vi "Connect.vi"(8 "error in (no error)":errorcluster, 10 "Addon Name":string, 11 "Address":string) -> (0 "error out":errorcluster, 3 "Ref":T1)   [LabVIEW 2019, in "Diagnostics Host Automation API.lvlib"]
uses:
  Diagnostics Host Automation API.lvlib
  Addon/Addon Shared/Types/HostAutomation.Ref.ctl
  <vilib>/NI/STM/TCP/TCP Connection Info.ctl
  <vilib>/NI/STM/SubVIs/MetaDataElement.ctl
  Addon/Addon Shared/Types/DTC.Codes.ctl
  <vilib>/NI/STM/TCP/Write Meta Data (TCP Ref).vi
  <vilib>/NI/STM/TCP/Write Meta Data (TCP Clst).vi
  <vilib>/NI/STM/NI STM.lvlib
  Addon/Addon Shared/Diagnostics Addon Shared.lvlib
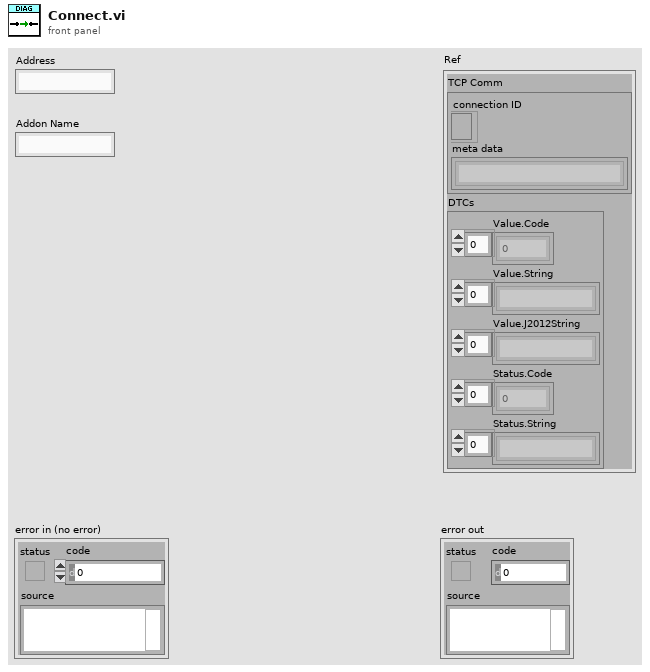
[diagram p1: front panel]
types:
  T1 = typedef "Diagnostics Addon Shared.lvlib/HostAutomation.Ref.ctl" = cluster{"TCP Comm":T2, "DTCs":T4}
  T2 = typedef "NI STM.lvlib/TCP Connection Info.ctl" = cluster{"connection ID":refnum<k5>, "meta data":T3[]}
  T3 = typedef "NI STM.lvlib/MetaDataElement.ctl" = string
  T4 = typedef "Diagnostics Addon Shared.lvlib/DTC.Codes.ctl" = cluster{"Value.Code":dbl[], "Value.String":string[], "Value.J2012String":string[], "Status.Code":dbl[], "Status.String":string[]}
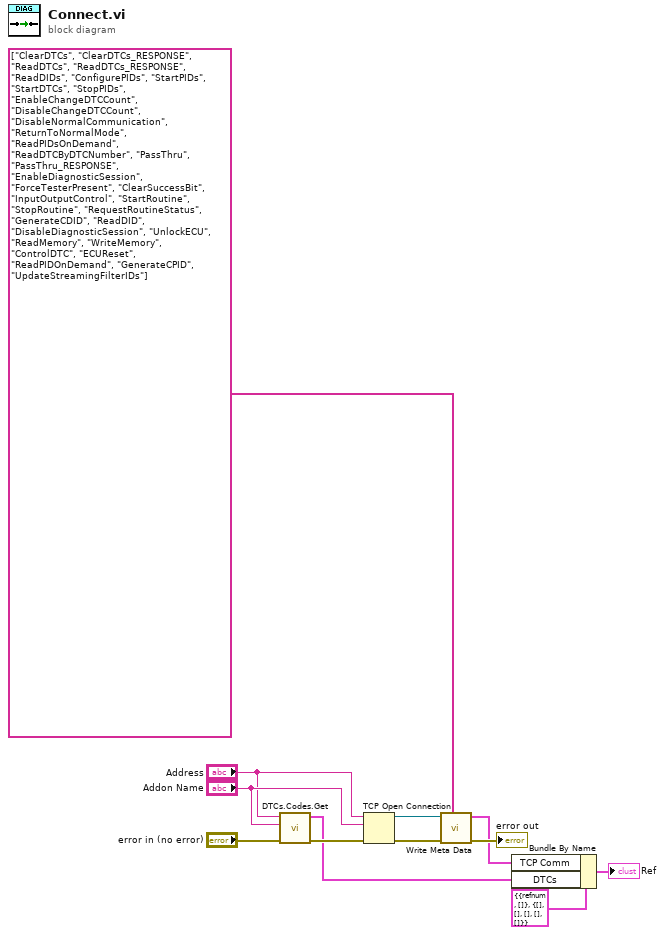
[diagram p0: block diagram]
diagram:
  n1 = call "DTCs.Codes.Get.vi"("error in (no error)"="error in (no error)", "Addon Name"="Addon Name", "Address"="Address") -> ("error out"=w6:errorcluster, "Codes"=w2:T4)  [unwired: 7 in]
  n2 = TCP Open Connection(address="Address", remote port or service name="Addon Name", error in (no error)=w6) -> (connection ID=w11:refnum<k5>, error out=w12:errorcluster)  [unwired: 2 in]
  n3 = call-poly <vilib>:"Write Meta Data.vi"("meta data"=string[] ["ClearDTCs", "ClearDTCs_RESPONSE", "ReadDTCs", "ReadDTCs_RESPONSE", "ReadDIDs", "ConfigurePIDs", "StartPIDs", "StartDTCs", "StopPIDs", "EnableChangeDTCCount", "DisableChangeDTCCount", "DisableNormalCommunication", "ReturnToNormalMode", "ReadPIDsOnDemand", "ReadDTCByDTCNumber", "PassThru", "PassThru_RESPONSE", "EnableDiagnosticSession", "ForceTesterPresent", "ClearSuccessBit", "InputOutputControl", "StartRoutine", "StopRoutine", "RequestRoutineStatus", "GenerateCDID", "ReadDID", "DisableDiagnosticSession", "UnlockECU", "ReadMemory", "WriteMemory", "ControlDTC", "ECUReset", "ReadPIDOnDemand", "GenerateCPID", "UpdateStreamingFilterIDs"] ("Meta data"), "error in"=w12, "connection ID"=w11) -> ("error out"=→"error out":errorcluster, "connection info out"=w3:T2)  [unwired: 7 in]
  n4 = Bundle By Name(cluster=T1 {"TCP Comm"={"connection ID"=refnum, "meta data"=[]}, "DTCs"={"Value.Code"=[], "Value.String"=[], "Value.J2012String"=[], "Status.Code"=[], "Status.String"=[]}} ("Ref"), "TCP Comm"=w3, "DTCs"=w2) -> (→"Ref":T1)
